vi "ThorLabs-Connect to Pinhole.vi"(8 "error in (no error)":errorcluster) -> (0 "error out":errorcluster, 3 "Thorlabs Pinhole Connected":bool)   [LabVIEW 2020]
uses:
  MPH_SDK/MPH16.lvlib
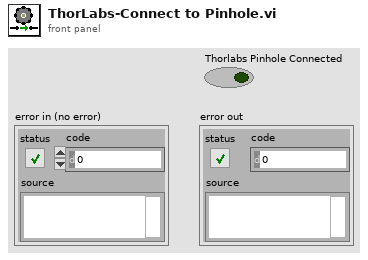
[diagram p1: front panel]
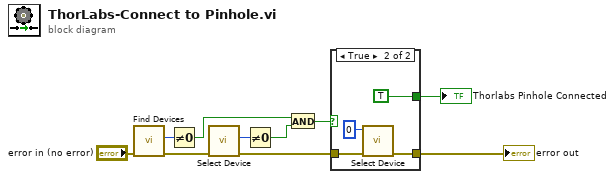
[diagram p0: block diagram]
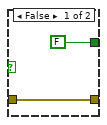
[diagram p2: hidden frame]
diagram:
  n1 = call "Find Devices.vi"("error in (no error)"="error in (no error)") -> ("error out"=w10:errorcluster, "function return"=w4:i32)  [unwired: 4 in, 1 out]
  n2 = Not Equal To 0?(x=w4) -> (x != 0?=w2:bool)
  n3 = call "Select Device.vi"("error in (no error)"=w10) -> ("error out"=w7:errorcluster, "function return"=w3:i32)  [unwired: 5 in]
  n4 = Not Equal To 0?(x=w3) -> (x != 0?=w1:bool)
  n5 = And(x=w2, y=w1) -> (x .and. y?=w8:bool)
  n6 = case shown="True" w8 {
    tunnel: w7 -> [w12 w15]
    tunnel: [w12 w14] -> w6
    tunnel: [FALSE TRUE] -> w5
    frame False {
    }
    frame True {
      n7 = call "Select Device.vi"("error in (no error)"=w15, "Device"=0 ("DeviceCount")) -> ("error out"=w14:errorcluster)  [unwired: 4 in, 1 out]
    }
  }
  "error out" <- w6
  "Thorlabs Pinhole Connected" <- w5
